vi "practice.vi"   [LabVIEW 2012, in "Mecanum Drive.lvrbt"]
uses:
  Mecanum Drive.lvrbt
  <vilib>/NXT/Hardware/Plugins/Tetrix DC Motor/TetrixDCMotorAddress.ctl
  <vilib>/NXT/NXTIO Xnodes/NXTIONodeSubVIs/TETRIX IO Check Battery.vi
  <vilib>/NXT/NXTIO Xnodes/NXTIONodeSubVIs/TETRIX IO Stop DC Motors.vi
  <vilib>/NXT/NXTIO Xnodes/NXTIONodeSubVIs/TETRIX IO Move DC Motors.vi
  <vilib>/NXT/NXTIO Xnodes/AddressXNode/NXTIOAddress.xnode
  <vilib>/NXT/NXTIO Xnodes/NXTIOXNode/NXTIO.xnode
  <vilib>/NXT/Subs/LVHSConnector.ctl
  <vilib>/NXT/LegoClasses/BrickReference/BrickReference.lvclass
types:
  T1 = typedef "TetrixDCMotorAddress.ctl" = i32
  T2 = cluster{"TetrixDCMotor":T1, "TetrixDCMotor 2":T1}
  T3 = typedef "LVHSConnector.ctl" = refnum<class "BrickReference.lvclass">
  T4 = typedef "FTC ControllerState.ctl" = cluster{"Left X":i8, "Left Y":i8, "Right X":i8, "Right Y":i8, "Button Encoding 9-12":u8, "Button Encoding 1-8":u8, "POV":T5}
  T5 = typedef "FTC POVState.ctl" = i8
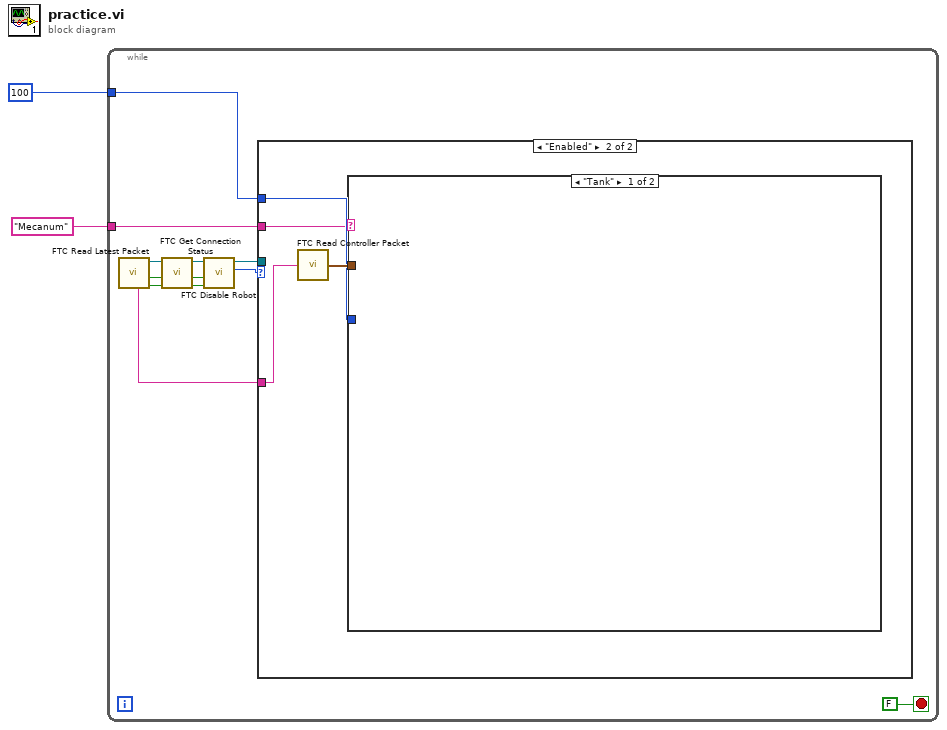
[diagram p0: block diagram]
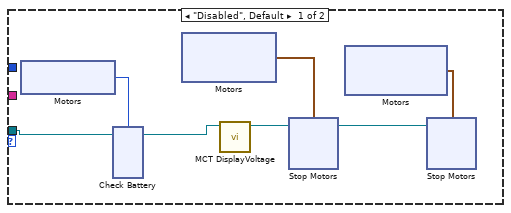
[diagram p2: hidden frame]
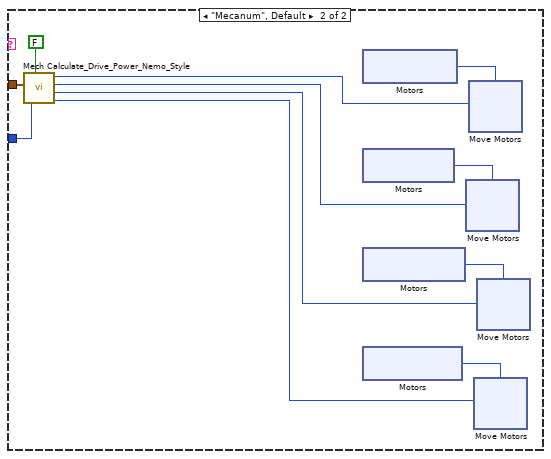
[diagram p3: hidden frame]
diagram:
  n1 = while {
    tunnel: 100 -> [w5]
    tunnel: "Mecanum" -> [w4]
    stop <- FALSE stop-if-true
    n2 = call <vilib>:"FTC Read Latest Packet.vi"() -> ("Packet Received?"=w14:bool, "Stopped?"=w12:bool, "NXT"=w13:T3, "Controller 1"=w8:string)  [unwired: 6 in, 2 out]
    n3 = call <vilib>:"FTC Get Connection Status.vi"("Packet Received?"=w14, "Stopped?"=w12, "NXT"=w13) -> ("Online?"=w9:bool, "Stopped?"=w10:bool, "NXT"=w11:T3)  [unwired: 5 in]
    n4 = call <vilib>:"FTC Disable Robot.vi"("Online?"=w9, "Stopped?"=w10, "NXT"=w11) -> ("Enabled?"=w7:enum16{"Disabled", "Enabled"}, "NXT"=w6:T3)  [unwired: 3 in]
    n5 = case shown="\"Enabled\"" w7 {
      tunnel: w8 -> [_ w42]
      tunnel: w6 -> [w21 _]
      tunnel: w5 -> [_ w41]
      tunnel: w4 -> [_ w40]
      frame "Disabled", Default {
        n6 = xnode "Motors"() -> ("Motor"=w15:T1)
        n7 = xnode "Check Battery"("Motors"=w15, "NXT/EV3"=w21) -> ("NXT/EV3"=w20:T3)  [unwired: 1 out]
        n8 = xnode "Motors"() -> ("Motor"=w16:cluster{"TetrixDCMotor":T1, "TetrixDCMotor":T1})
        n9 = call <vilib>:"MCT DisplayVoltage.vi"("NXT"=w20) -> ("NXT"=w19:T3)  [unwired: 10 in]
        n10 = xnode "Stop Motors"("Motors"=w16, "NXT/EV3"=w19) -> ("NXT/EV3"=w18:T3)
        n11 = xnode "Motors"() -> ("Motor"=w17:cluster{"TetrixDCMotor":T1, "TetrixDCMotor":T1})
        n12 = xnode "Stop Motors"("Motors"=w17, "NXT/EV3"=w18) -> ()  [unwired: 1 out]
      }
      frame "Enabled" {
        n13 = call <vilib>:"FTC Read Controller Packet.vi"("Packet"=w42) -> ("Controller State"=w43:T4)  [unwired: 4 in]
        n14 = case shown="\"Tank\"" w40 {
          tunnel: w43 -> [_ w50]
          tunnel: w41 -> [_ w45]
          frame "Tank" {
          }
          frame "Mecanum", Default {
            n15 = call "Mech Calculate_Drive_Power_Nemo_Style.vi"("Power"=w45, "Reverse"=FALSE, "Controller State"=w50) -> ("Right Rear Power"=w46:i8, "Right Front Power"=w47:i8, "Left Rear Power"=w48:i8, "Left Front Power"=w49:i8)  [unwired: 5 in]
            n16 = xnode "Motors"() -> ("Motor"=w54:T1)
            n17 = xnode "Motors"() -> ("Motor"=w52:T1)
            n18 = xnode "Motors"() -> ("Motor"=w51:T1)
            n19 = xnode "Motors"() -> ("Motor"=w53:T1)
            n20 = xnode "Move Motors"("Power/Speed 1"=w48, "Motors"=w52) -> ()  [unwired: 1 in, 1 out]
            n21 = xnode "Move Motors"("Power/Speed 1"=w49, "Motors"=w54) -> ()  [unwired: 1 in, 1 out]
            n22 = xnode "Move Motors"("Power/Speed 1"=w46, "Motors"=w53) -> ()  [unwired: 1 in, 1 out]
            n23 = xnode "Move Motors"("Power/Speed 1"=w47, "Motors"=w51) -> ()  [unwired: 1 in, 1 out]
          }
        }
      }
    }
  }
